vi "OAT Compensate Vector Data (N Channels).vi"(0 "magnitudes [RMS]":T2(array[cluster]) {"magnitude" format="%.2f"; "time/rev/rpm" format="%.2f"}, 2 "reset? (F)":bool, 5 "phases [phase lag]":cluster{"time/rev/rpm":dbl[], "phase":dbl[]}[][](array[cluster]) {"phase" format="%.2f"; "time/rev/rpm" format="%.2f"}, 7 "vector references":cdb[][](array[numeric]) format="%.2f", 11 "error in (no error)":errorcluster, 13 "view info":T1={"dB on? (F)"=FALSE, "unwrap phase? (T)"=TRUE, "unit in degree? (T)"=TRUE}) -> (4 "compensated magnitudes [RMS]":T2(array[cluster]) {"magnitude" format="%.2f"; "time/rev/rpm" format="%.2f"}, 6 "compensated phases [phase lag]":cluster{"time/rev/rpm":dbl[], "phase":dbl[]}[][](array[cluster]) {"phase" format="%.2f"; "time/rev/rpm" format="%.2f"}, 8 "actual vector references":cdb[][](array[numeric]) format="%.2f", 15 "error out":errorcluster)   [LabVIEW 2017, in "SoundVib_RefDataProcess.lvlib"]
doc: "Compensates for the shaft bow and electrical variations in displacement transducer signals. This VI performs slow-roll compensation by subtracting <B>vector references</B> from the corresponding <B>magnitudes [RMS]</B> and <B>phases [phase lag]</B>. Wire data to the <B>magnitudes [RMS]</B> and <B>phases [phase lag]</B> inputs to determine the polymorphic instance to use or manually select the instance."
uses:
  <vilib>/addons/Sound and Vibration/Order Analysis/Referece Data Processing/SoundVib_RefDataProcess.lvlib
  <vilib>/addons/Sound and Vibration/Order Analysis/Misc/OAT Convert Phase (N Channels).vi
  <vilib>/Analysis/NI_AALPro.lvlib
  <vilib>/addons/Sound and Vibration/Order Analysis/Resample Order Tracking/SoundVib_Resampling.lvlib
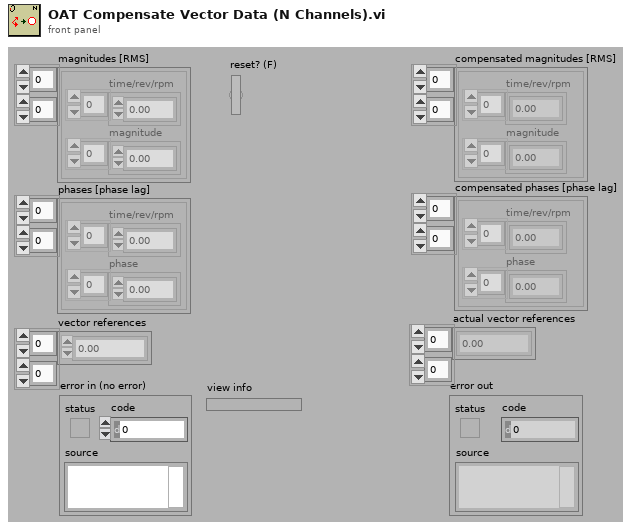
[diagram p1: front panel]
types:
  T1 = cluster{"dB on? (F)":bool, "unwrap phase? (T)":bool, "unit in degree? (T)":bool}
  T2 = cluster{"time/rev/rpm":dbl[], "magnitude":dbl[]}[][]
  T3 = cluster{"unwrap phase? (T)":bool, "unit in degree? (T)":bool}
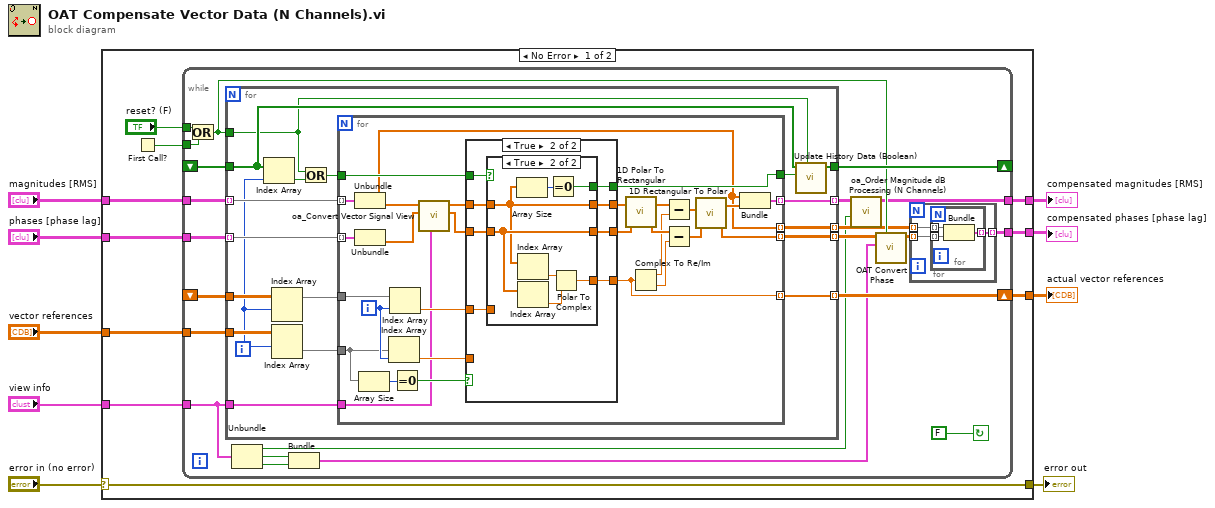
[diagram p0: block diagram]
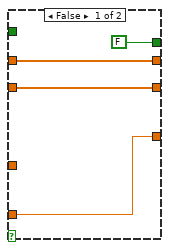
[diagram p2: hidden frame]
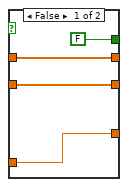
[diagram p3: hidden frame]
diagram:
  n1 = case shown="No Error" "error in (no error)" {
    selector: "error in (no error)" -> [w10 w121]
    tunnel: "magnitudes [RMS]" -> [w12 w120]
    tunnel: "phases [phase lag]" -> [w19 w119]
    tunnel: "vector references" -> [w15 w118]
    tunnel: [w18 w120] -> w6
    tunnel: [w11 w119] -> w5
    tunnel: [w10 w121] -> w3
    tunnel: [w17 w118] -> w2
    tunnel: "view info" -> [w16 _]
    frame No Error {
      n2 = First Call?() -> (First Call?: T/F=w14:bool)
      n3 = while {
        tunnel: w12 -> [w40]
        tunnel: w19 -> [w39]
        tunnel: [w21] -> w18
        shift-right: [w38] -> w17
        shift-left: _ -> [w37]
        tunnel: w16 -> [w26]
        tunnel: w15 -> [w36]
        shift-right: [w34] -> _
        shift-left: _ -> [w35]
        tunnel: w14 -> [w31]
        tunnel: "reset? (F)" -> [w32]
        tunnel: [w27] -> w11
        stop <- FALSE continue-if-true
        n4 = Or(x=w32, y=w31) -> (x .or. y?=w30:bool)
        n5 = for {
          tunnel: [w48] -> w22 mode=indexing
          tunnel: w40 -> [w65] mode=indexing
          tunnel: w39 -> [w64] mode=indexing
          tunnel: [w63] -> w38 mode=indexing
          tunnel: w37 -> [w61]
          tunnel: w26 -> [w62]
          tunnel: w36 -> [w59]
          tunnel: w35 -> [w55]
          tunnel: [w56] -> w34
          tunnel: [w51] -> w29 mode=indexing
          tunnel: [w50] -> w33 mode=indexing
          tunnel: w30 -> [w49]
          i -> [w52]
          n6 = Index Array(array=w55, index=w52) -> (element=w54:bool)
          n7 = Index Array(array=w61, index (row)=w52) -> (element=w60:cdb[])  [unwired: 1 in]
          n8 = Index Array(array=w59, index (row)=w52) -> (element=w58:cdb[])  [unwired: 1 in]
          n9 = Or(x=w49, y=w54) -> (x .or. y?=w53:bool)
          n10 = for {
            tunnel: w65 -> [w94] mode=indexing
            tunnel: w64 -> [w93] mode=indexing
            tunnel: [w92] -> w48 mode=indexing
            tunnel: [w81] -> w63 mode=indexing
            tunnel: w60 -> [w80]
            tunnel: w53 -> [w91]
            tunnel: w62 -> [w66]
            tunnel: w58 -> [w71]
            tunnel: [w76] -> w57
            tunnel: [w75] -> w51 mode=indexing
            tunnel: [w74] -> w50 mode=indexing
            i -> [w78]
            n11 = Unbundle(w94) -> ("time/rev/rpm"=w75:dbl[], "magnitude"=w70:dbl[])
            n12 = Unbundle(w93) -> ("phase"=w68:dbl[])  [unwired: 1 out]
            n13 = Array Size(array=w71) -> (size(s)=w73:i32)
            n14 = Index Array(array=w71, index=w78) -> (element=w77:cdb)
            n15 = Index Array(array=w80, index=w78) -> (element=w79:cdb)
            n16 = Equal To 0?(x=w73) -> (x = 0?=w72:bool)
            n17 = call <vilib>:"oa_Convert Vector Signal View.vi"("view"=w66, "phase"=w68, "magnitude"=w70) -> ("phase out"=w67:dbl[], "magnitude out"=w69:dbl[])  [unwired: 7 in]
            n18 = case shown="True" w72 {
              tunnel: w91 -> [_ w106]
              tunnel: w69 -> [w96 w105]
              tunnel: [w96 w104] -> w90
              tunnel: [w97 w103] -> w89
              tunnel: w67 -> [w97 w102]
              tunnel: [w98 w101] -> w81
              tunnel: w79 -> [_ w100]
              tunnel: w77 -> [w98 _]
              tunnel: [FALSE w99] -> w76
              frame False {
              }
              frame True {
                n19 = case shown="True" w106 {
                  tunnel: w105 -> [w109 w113]
                  tunnel: [w110 w114] -> w101
                  tunnel: w102 -> [w108 w117]
                  tunnel: w100 -> [w110 _]
                  tunnel: [w109 w113] -> w104
                  tunnel: [w108 w117] -> w103
                  tunnel: [FALSE w111] -> w99
                  frame False {
                  }
                  frame True {
                    n20 = Array Size(array=w113) -> (size(s)=w112:i32)
                    n21 = Index Array(array=w113) -> (element=w116:dbl)  [unwired: 1 in]
                    n22 = Index Array(array=w117) -> (element=w115:dbl)  [unwired: 1 in]
                    n23 = Equal To 0?(x=w112) -> (x = 0?=w111:bool)
                    n24 = Polar To Complex(1:w115, 2:w116) -> (0:w114:cdb)
                  }
                }
              }
            }
            n25 = call <vilib>:"1D Polar To Rectangular.vi"("Magnitude"=w90, "Phase"=w89) -> ("X"=w88:dbl[], "Y"=w87:dbl[])  [unwired: 1 out]
            n26 = Complex To Re/Im(x + iy=w81) -> (x=w83:dbl, y=w82:dbl)
            n27 = Subtract(x=w88, y=w83) -> (x-y=w86:dbl[])
            n28 = Subtract(x=w87, y=w82) -> (x-y=w85:dbl[])
            n29 = call <vilib>:"1D Rectangular To Polar.vi"("X"=w86, "Y"=w85) -> ("Magnitude"=w84:dbl[], "Phase"=w74:dbl[])  [unwired: 1 out]
            n30 = Bundle("time/rev/rpm"=w75, "Magnitude"=w84) -> (w92:cluster{"time/rev/rpm":dbl[], "Magnitude":dbl[]})  [unwired: 1 in]
          }
          n31 = call <vilib>:"Update History Data (Boolean).vi"("reset?"=w49, "new data"=w57, "History Data In"=w55) -> ("History Data Out"=w56:bool[])  [unwired: 8 in]
        }
        n32 = Unbundle(w26) -> ("dB on? (F)"=w20:bool, "unwrap phase? (T)"=w25:bool, "unit in degree? (T)"=w24:bool)
        n33 = Bundle("unwrap phase? (T)"=w25, "unit in degree? (T)"=w24) -> (w23:T3)  [unwired: 1 in]
        n34 = call <vilib>:"oa_Order Magnitude dB Processing (N Channels).vi"("dB on? (T)"=w20, "magnitudes"=w22) -> ("magnitudes dB"=w21:cluster{"X":dbl[], "Y":dbl[]}[][])  [unwired: 9 in]
        n35 = call-poly <vilib>:"OAT Convert Phase.vi"("reset (TRUE)"=w30, "desired phase setting"=w23, "phase in"=w33) -> ("phase out"=w28:dbl[][][])  [unwired: 8 in]
        n36 = for {
          tunnel: w29 -> [w44] mode=indexing
          tunnel: w28 -> [w43] mode=indexing
          tunnel: [w42] -> w27 mode=indexing
          n37 = for {
            tunnel: w44 -> [w46] mode=indexing
            tunnel: w43 -> [w47] mode=indexing
            tunnel: [w45] -> w42 mode=indexing
            n38 = Bundle("time/rev/rpm"=w46, "phase out"=w47) -> (w45:cluster{"time/rev/rpm":dbl[], "phase out":dbl[]})  [unwired: 1 in]
          }
        }
      }
    }
    frame Error {
    }
  }
  "error out" <- w3
  "compensated magnitudes [RMS]" <- w6
  "compensated phases [phase lag]" <- w5
  "actual vector references" <- w2
